vi "Construct Text Log Sink.vi"(7 "LogLevel":T1, 10 "File Name":string, 11 "Log File Folder":path) -> (3 "Text File Sink out":refnum<class "Text File Sink.lvclass">)   [LabVIEW 2017, in "Text File Sink.lvclass"]
doc: "Construct an instance of text log sink. If no file name is input, the file name will be 'Application Directory Name Event Log'. If no log file folder is input, the log file folder will be Public Application Data\\Application Directory Name Event Logs. \n - File extension used is .txt. \n - File will be rolled over at 1Mb.\n - File name will include a timestamp when that file was created.\nFor control over these default values, use the advanced constructor."
uses:
  <vilib>/gpm_packages/@cs/event-logger/Source/Text File Sink/Text File Sink.lvclass
  C:/Program Files/National Instruments/LabVIEW 2017/vi.lib/gpm_packages/@cs/event-logger/Source/Composed Log/Log Sink/Log Sink.lvclass
  <vilib>/gpm_packages/@cs/event-logger/Source/Composed Log/Types/Log Level.ctl
  <vilib>/gpm_packages/@cs/event-logger/Source/Text File Sink/Configuration.ctl
  <vilib>/Utility/sysdir.llb/System Directory Type.ctl
  <vilib>/gpm_packages/@cs/event-logger/Source/Text File Sink/Text File Sink.lvclass/Text File Sink.ctl
  <vilib>/gpm_packages/@cs/event-logger/Source/Composed Log/Log Sink/Log Sink.lvclass/Log Sink.ctl
  <vilib>/gpm_packages/@cs/event-logger/Source/Composed Log/Log Sink/Log Sink.lvclass
  <vilib>/gpm_packages/@cs/event-logger/Source/Composed Log/Composed Log.lvlib
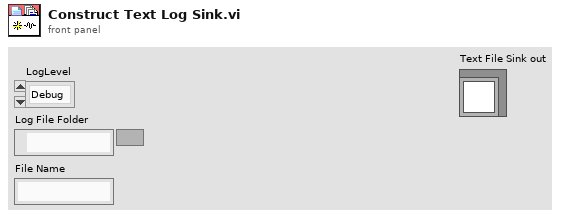
[diagram p1: front panel]
types:
  T1 = typedef "Composed Log.lvlib/Log Level.ctl" = enum16{"Debug", "Info", "Warning", "Error", "Critical"}
  T2 = typedef "Text File Sink.lvclass/Configuration.ctl" = cluster{"Folder":path, "Name":string, "Extension":string, "Max Size (MB)":i64, "Timestamp Filename":bool}
  T3 = typedef "System Directory Type.ctl" = i32
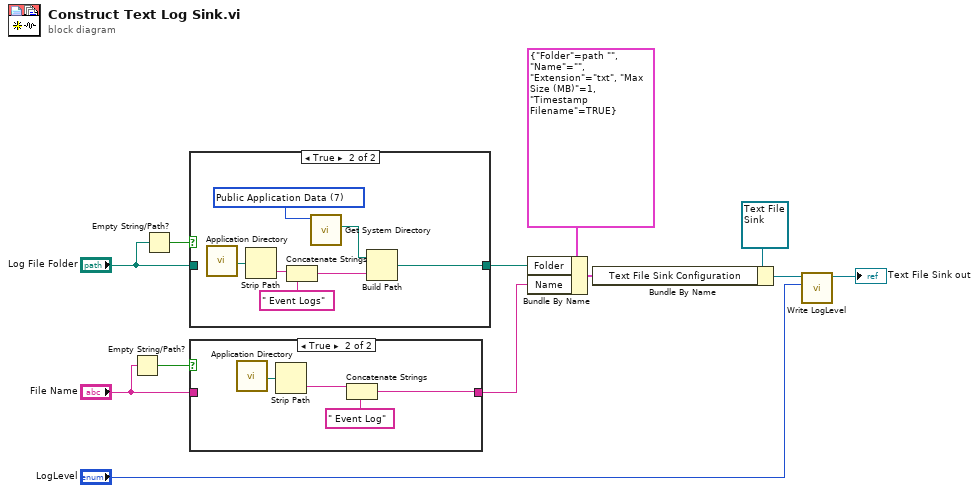
[diagram p0: block diagram]
diagram:
  n1 = Empty String/Path?(string/path="File Name") -> (empty?=w4:bool)
  n2 = Empty String/Path?(string/path="Log File Folder") -> (empty?=w7:bool)
  n3 = case shown="True" w7 {
    tunnel: "Log File Folder" -> [w13 _]
    tunnel: [w13 w14] -> w5
    frame False {
    }
    frame True {
      w20 = T3 7 items=["User Home"=0, "User Desktop"=1, "User Documents"=2, "User Application Data"=3, "User Preferences"=4, "User Temporary"=5, "Public Documents"=6, "Public Application Data"=7, "Public Preferences"=8, "Public Cache"=13, "System Core Libraries"=9, "System Installed Libraries"=10, "Application Files"=11, "Boot Volume Root"=12] ("system directory type")
      n4 = call <vilib>:"Application Directory.vi"() -> ("Application Directory"=w19:path)
      n5 = Strip Path(path=w19) -> (name=w18:string)  [unwired: 1 out]
      n6 = Concatenate Strings(w18, " Event Logs" ("string")) -> (w16:string)
      n7 = call <vilib>:"Get System Directory.vi"("system directory type"=w20) -> ("system directory"=w15:path)  [unwired: 10 in]
      n8 = Build Path(base path=w15, name or relative path=w16) -> (appended path=w14:path)
    }
  }
  n9 = case shown="True" w4 {
    tunnel: "File Name" -> [w21 _]
    tunnel: [w21 w22] -> w2
    frame False {
    }
    frame True {
      n10 = call <vilib>:"Application Directory.vi"() -> ("Application Directory"=w25:path)
      n11 = Strip Path(path=w25) -> (name=w24:string)  [unwired: 1 out]
      n12 = Concatenate Strings(w24, " Event Log" ("string")) -> (w22:string)
    }
  }
  n13 = Bundle By Name(cluster=T2 {"Folder"=path "", "Name"="", "Extension"="txt", "Max Size (MB)"=1, "Timestamp Filename"=TRUE} ("Text File Sink Configuration"), "Folder"=w5, "Name"=w2) -> (w8:T2)
  n14 = Bundle By Name(cluster=refnum<class "Text File Sink.lvclass"> refnum ("Text File Sink in"), "Text File Sink Configuration"=w8) -> (w1:refnum<class "Text File Sink.lvclass">)
  n15 = call <vilib>:"Write LogLevel.vi"("LogLevel"="LogLevel", "Log Sink in"=w1) -> ("Log Sink out"=→"Text File Sink out":refnum<class "Text File Sink.lvclass">)  [unwired: 8 in, 1 out]
